vi "4.3.vi"(1 "数值":dbl) -> (0 "平均值":dbl)   [LabVIEW 2017]
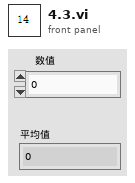
[diagram p1: front panel]
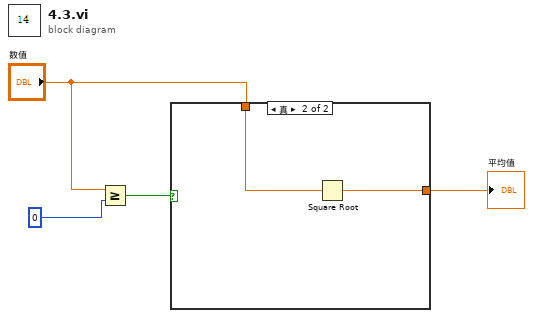
[diagram p0: block diagram]
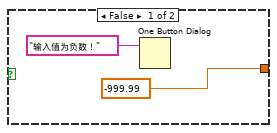
[diagram p2: hidden frame]
diagram:
  n1 = Greater Or Equal?(x="数值", y=0) -> (x >= y?=w3:bool)
  n2 = case shown="真" w3 {
    tunnel: "数值" -> [_ w8]
    tunnel: [-999.99 w7] -> w4
    frame False {
      n3 = One Button Dialog(message="输入值为负数！") -> ()  [unwired: 1 in, 1 out]
    }
    frame True {
      n4 = Square Root(x=w8) -> (sqrt(x)=w7:dbl)
    }
  }
  "平均值" <- w4
